vi "sort 1D array (SubVI).vi"(10 "order":i32[](array[numeric]), 11 "Array in":dbl[](array[numeric])) -> (3 "Array out":dbl[](array[numeric]))   [LabVIEW 2024]
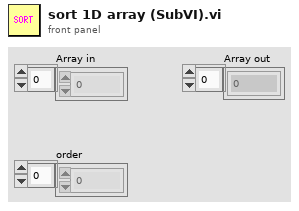
[diagram p1: front panel]
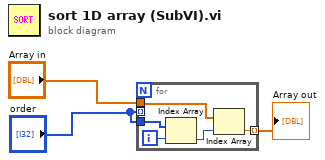
[diagram p0: block diagram]
diagram:
  n1 = for {
    tunnel: "order" -> [_] mode=indexing
    tunnel: "order" -> [w7]
    tunnel: "Array in" -> [w5]
    tunnel: [w4] -> w3 mode=indexing
    i -> [w8]
    n2 = Index Array(array=w7, index=w8) -> (element=w6:i32)
    n3 = Index Array(array=w5, index=w6) -> (element=w4:dbl)
  }
  "Array out" <- w3
